vi "fiboacci_iterative.vi"(9 "n":u8, 10 "b":dbl, 11 "a":dbl=1.0) -> (1 "F(n)":dbl)   [LabVIEW 2021]
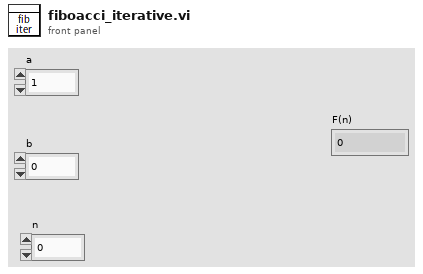
[diagram p1: front panel]
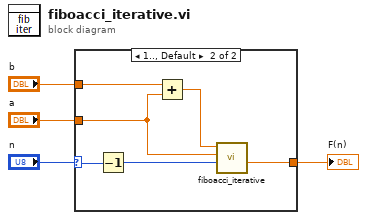
[diagram p0: block diagram]
diagram:
  n1 = case shown="1.., Default" "n" {
    selector: "n" -> [_ w7]
    tunnel: "b" -> [w5 w11]
    tunnel: "a" -> [_ w9]
    tunnel: [w5 w8] -> w2
    frame 0 {
    }
    frame 1.., Default {
      n2 = Decrement(x=w7) -> (x-1=w6:u8)
      n3 = Add(x=w11, y=w9) -> (x+y=w10:dbl)
      n4 = call "fiboacci_iterative.vi"("n"=w6, "b"=w9, "a"=w10) -> ("F(n)"=w8:dbl)  [unwired: 8 in]
    }
  }
  "F(n)" <- w2
